vi "checkStiffnessOutOfRange.vi"(8 "error in (no error)":errorcluster, 11 "Model in":refnum<class "Model.lvclass">) -> (0 "error out":errorcluster, 2 "stiffnessOutOfRangeIsTrue":bool, 3 "Model out":refnum<class "Model.lvclass">)   [LabVIEW 2013, in "Model.lvclass"]
uses:
  Model.lvclass
  Model.lvclass/Model.ctl
  ApplicationElements/StiffnessMonitor/StiffnessMonitor.lvclass
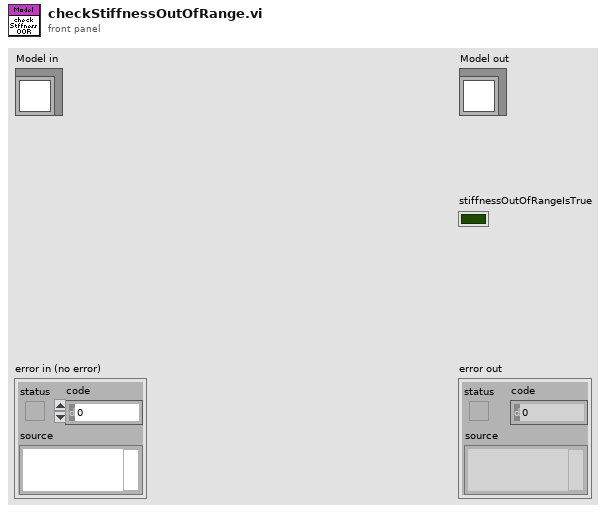
[diagram p1: front panel]
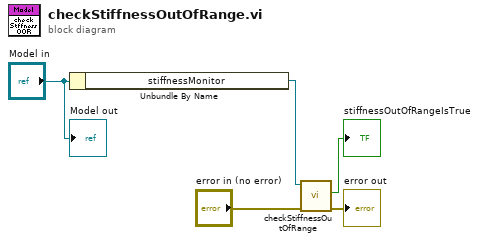
[diagram p0: block diagram]
diagram:
  n1 = Unbundle By Name("Model in") -> ("stiffnessMonitor"=w4:refnum<class "StiffnessMonitor.lvclass">)
  n2 = call "checkStiffnessOutOfRange.vi"("error in (no error)"="error in (no error)", "StiffnessMonitor in"=w4) -> ("error out"=→"error out":errorcluster, "stiffnessOutOfRangeIsTrue"=→"stiffnessOutOfRangeIsTrue":bool)  [unwired: 7 in, 1 out]
  "Model out" <- "Model in"
